vi "Wall_Tunneling.vi"(6 "Tunnal All (F)":bool, 10 "Walls to Tunnel":i32=2, 11 "Line to Parse":u32[](array[numeric]) format="%06x") -> (1 "Tile Type":u16[](array[ring]), 2 "Array":T1[](array[typedef]) {"R" format="%.0x"; "G" format="%.0x"; "B" format="%.0x"}, 3 "Wall Index":i32[](array[numeric]), 4 "Wall Thickness (px)":i32)   [LabVIEW 2016]
doc: "<B>Description:</B> Tunnels through the specified number of walls. Retuns the the index where the wall ends. If <B>Walls to Tunnel</B> = 1, also returns correct information on the thickness of the walls.\n\n<B>Date:</B> 1/2019\n<B>Author:</B> Luke Jarocki, Choose Movement Consulting, LLC"
uses:
  Controls/Split_Color.ctl
panel:
  out "Array 2":cluster{i32, bool, "IsWhiteSpace":u16}[](array[cluster])
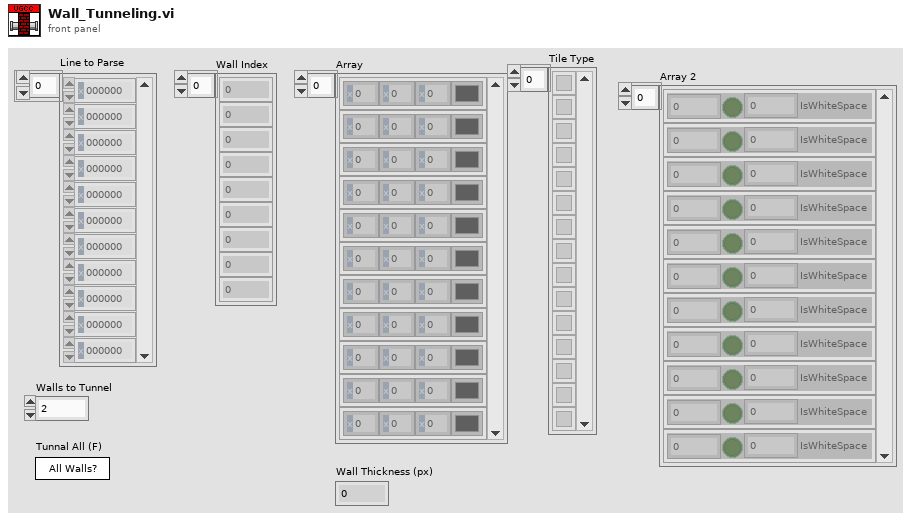
[diagram p1: front panel]
types:
  T1 = typedef "Split_Color.ctl" = cluster{"R":u8, "G":u8, "B":u8, "Color Box":u32}
  T2 = typedef "TileColor.ctl" = u16
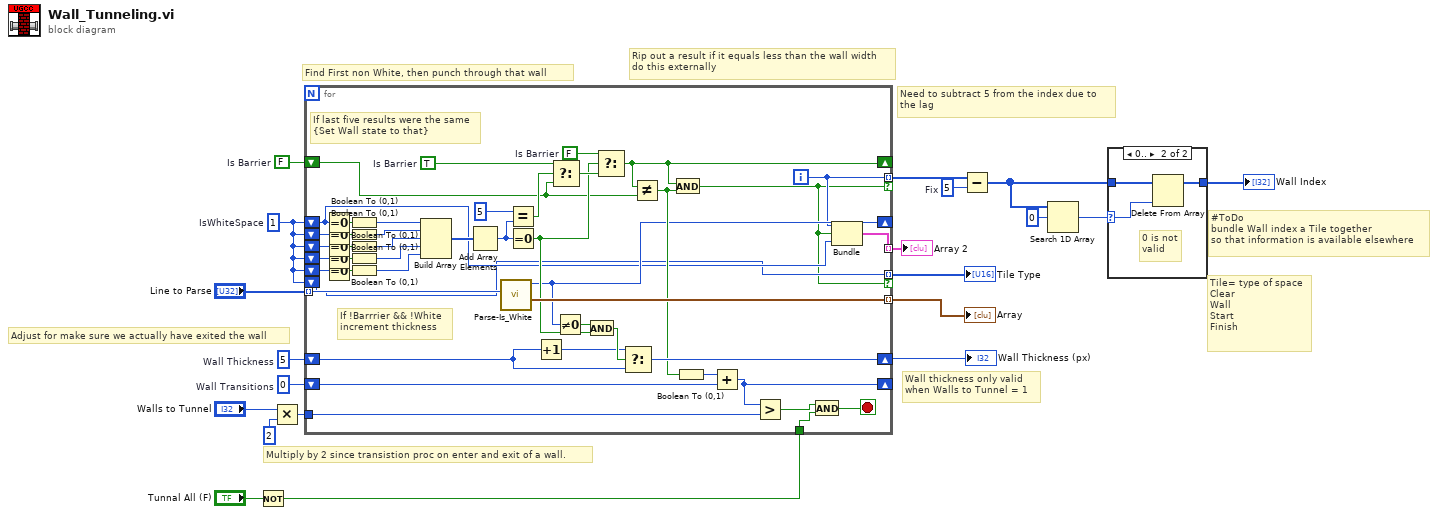
[diagram p0: block diagram]
diagram:
  w1 = u16 1  # IsWhiteSpace
  w10 = 5  # Fix
  w16 = 0  # Wall Transitions
  w17 = FALSE  # Is Barrier
  w20 = 5  # Wall Thickness
  # "Tile= type of space\nClear\nWall\nStart\nFinish"
  # "#ToDo\nbundle Wall index a Tile together\nso that information is available elsewhere"
  # "Multiply by 2 since transistion proc on enter and exit of a wall."
  # "Need to subtract 5 from the index due to\nthe lag"
  # "Rip out a result if it equals less than the wall width\ndo this externally"
  # "Wall thickness only valid\nwhen Walls to Tunnel = 1"
  # "Adjust for make sure we actually have exited the wall"
  # "Find First non White, then punch through that wall"
  n1 = Not(x="Tunnal All (F)") -> (.not. x?=w8:bool)
  n2 = Multiply(x="Walls to Tunnel", y=2) -> (x*y=w13:i32)
  n3 = for {
    tunnel: "Line to Parse" -> [w65] mode=indexing
    shift-right: [w26] -> _
    shift-left: w1 -> [w24]
    tunnel: [w64] -> w18 mode=indexing
    tunnel: [w22] -> w19 mode=indexing if=w21
    shift-right: [w63] -> w12
    shift-left: w20 -> [w54]
    tunnel: [w25] -> w11 mode=indexing if=w21
    tunnel: w13 -> [w47]
    shift-left: w1 -> [w30]
    shift-left: w1 -> [w28]
    shift-left: w1 -> [w29]
    shift-left: w1 -> [w27]
    shift-right: [w44] -> _
    shift-left: w17 -> [w46]
    shift-right: [w48] -> _
    shift-left: w16 -> [w49]
    tunnel: w8 -> [w42]
    tunnel: [w23] -> w2 mode=indexing
    shift-left: w1 -> [w22]
    i -> [w25]
    stop <- w41 stop-if-true
    w59 = FALSE  # Is Barrier
    w60 = TRUE  # Is Barrier
    # "If last five results were the same\n{Set Wall state to that}"
    # "If !Barrrier && !White\nincrement thickness"
    n4 = Equal To 0?(x=w24) -> (x = 0?=w40:bool)
    n5 = Equal To 0?(x=w30) -> (x = 0?=w38:bool)
    n6 = Equal To 0?(x=w28) -> (x = 0?=w36:bool)
    n7 = Equal To 0?(x=w29) -> (x = 0?=w35:bool)
    n8 = Equal To 0?(x=w27) -> (x = 0?=w34:bool)
    n9 = Boolean To (0,1)(Boolean=w40) -> (0, 1=w39:i16)
    n10 = Boolean To (0,1)(Boolean=w38) -> (0, 1=w37:i16)
    n11 = Boolean To (0,1)(Boolean=w36) -> (0, 1=w33:i16)
    n12 = Boolean To (0,1)(Boolean=w35) -> (0, 1=w32:i16)
    n13 = Boolean To (0,1)(Boolean=w34) -> (0, 1=w31:i16)
    n14 = Build Array(w39, w37, w33, w32, w31) -> (w61:i16[])
    n15 = Add Array Elements(numeric array=w61) -> (sum=w57:i16)
    n16 = call "Parse-Is_White.vi"("Color"=w65) -> ("Color Cluster"=w64:T1, "Tile Color"=w26:T2)  [unwired: 8 in, 1 out]
    n17 = Equal?(x=u32 5, y=w57) -> (x = y?=w53:bool)
    n18 = Equal To 0?(x=w57) -> (x = 0?=w52:bool)
    n19 = Increment(x=w54) -> (x+1=w55:i32)
    n20 = Select(t=w60, s=w53, f=w46) -> (s? t:f=w58:bool)
    n21 = Not Equal To 0?(x=w26) -> (x != 0?=w51:bool)
    n22 = And(x=w51, y=w52) -> (x .and. y?=w56:bool)
    n23 = Select(t=w59, s=w52, f=w58) -> (s? t:f=w44:bool)
    n24 = Select(t=w55, s=w56, f=w54) -> (s? t:f=w63:i32)
    n25 = Not Equal?(x=w44, y=w46) -> (x != y?=w45:bool)
    n26 = And(x=w44, y=w45) -> (x .and. y?=w21:bool)
    n27 = Boolean To (0,1)(Boolean=w45) -> (0, 1=w50:i16)
    n28 = Add(x=w50, y=w49) -> (x+y=w48:i32)
    n29 = Greater?(x=w48, y=w47) -> (0:w43:bool)
    n30 = And(x=w43, y=w42) -> (x .and. y?=w41:bool)
    n31 = Bundle(w25, w21, "Tile Color"=w24) -> (w23:cluster{i32, bool, "Tile Color":T2})  [unwired: 1 in]
  }
  "Array" <- w18
  "Wall Thickness (px)" <- w12
  "Tile Type" <- w19
  "Array 2" <- w2
  n32 = Subtract(x=w11, y=w10) -> (x-y=w5:i32[])
  n33 = Search 1D Array(1D array=w5, element=0) -> (index of element=w6:i32)  [unwired: 1 in]
  n34 = case shown="0.." w6 {
    selector: w6 -> [_ w67]
    tunnel: [w66 w68] -> w4
    tunnel: w5 -> [w66 w69]
    frame ..-1, Default {
    }
    frame 0.. {
      # "0 is not\nvalid"
      n35 = Delete From Array(array=w69, index=w67) -> (array with subset deleted=w68:i32[])  [unwired: 1 in, 1 out]
    }
  }
  "Wall Index" <- w4
